vi "Get Timing.vi"(8 "error in (no error)":errorcluster, 11 "RP I-V Driver in":refnum<class "RP I-V Driver.lvclass">) -> (0 "error out":errorcluster, 1 "Decimation":i32=1, 2 "Rate":dbl=125000000.0 format="%#_6pHz", 3 "RP I-V Driver out":refnum<class "RP I-V Driver.lvclass">)   [LabVIEW 2024, in "RP I-V Driver.lvclass"]
uses:
  RP I-V Driver.lvclass
  D:/GitHub/NHMFL_Core/Libraries/Red Pitaya/Red Pitaya Digitizer/Red Pitaya Digitizer.lvclass
  Red Pitaya Digitizer/Red Pitaya Digitizer.lvclass/Red Pitaya Digitizer.ctl
  Red Pitaya Digitizer/Read Logic tag.vi
  Red Pitaya Digitizer/Red Pitaya Digitizer.lvclass
  RP I-V Driver.lvclass/RP I-V Driver.ctl
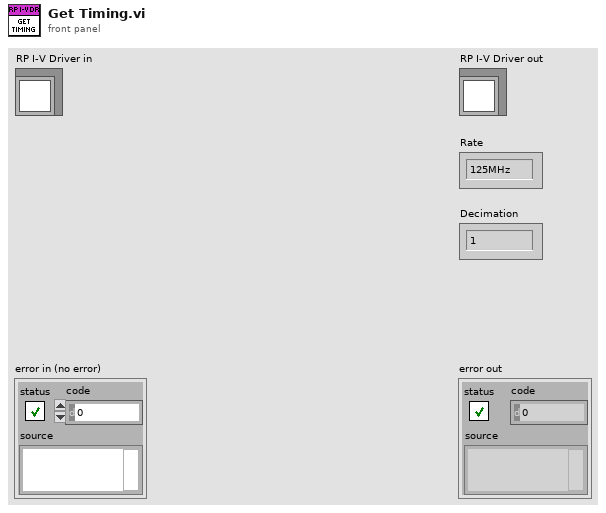
[diagram p1: front panel]
types:
  T1 = typedef "RP I-V Configuration.ctl" = cluster{"I-V parameters":T2, "Ranges":dbl[], "Post-trigger delay":dbl, "Post-trigger duration":dbl, "Output delay":dbl}
  T2 = typedef "I-V parameters.ctl" = cluster{"Start magnitude":dbl, "Magnitude increment":dbl, "End magnitude":dbl, "Ramp length":i32, "Top  length":i32, "Threshold ":dbl, "Processing delay":u16, "Output gain ":dbl, "Interpolation":i32, "Stop after":u16, "Detector window":i32}
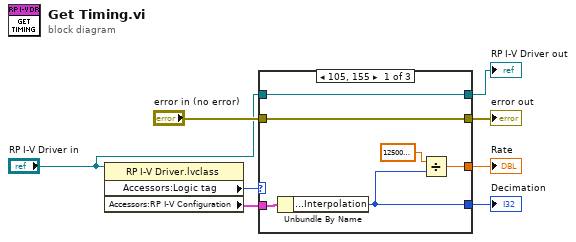
[diagram p0: block diagram]
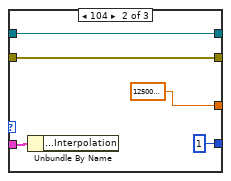
[diagram p2: hidden frame]
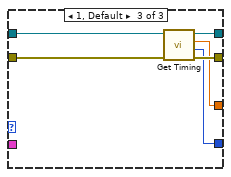
[diagram p3: hidden frame]
diagram:
  n1 = property class="RP I-V Driver.lvclass"(reference="RP I-V Driver in") -> ("Accessors:Logic tag"=w2:u16, "Accessors:RP I-V Configuration"=w1:T1)  [unwired: 1 in, 2 out]
  n2 = case shown="105, 155" w2 {
    tunnel: [w10 w18 w25] -> w8
    tunnel: [w11 1 ("Decimation") w24] -> w7
    tunnel: [w12 125000000.0 ("y") w23] -> w6
    tunnel: [w9 w17 w22] -> w5
    tunnel: "error in (no error)" -> [w10 w18 w21]
    tunnel: "RP I-V Driver in" -> [w9 w17 w20]
    tunnel: w1 -> [w14 w19 _]
    frame 105, 155 {
      n3 = Unbundle By Name(w14) -> ("I-V parameters.Interpolation"=w11:i32)
      n4 = Divide(x=125000000.0 ("y"), y=w11) -> (x/y=w12:dbl)
    }
    frame 104 {
      n5 = Unbundle By Name(w19) -> ()  [unwired: 1 out]
    }
    frame 1, Default {
      n6 = call-parent "Get Timing.vi"("error in (no error)"=w21, "Red Pitaya Digitizer in"=w20) -> ("error out"=w25:errorcluster, "Decimation"=w24:i32, "Rate"=w23:dbl, "Red Pitaya Digitizer out"=w22:refnum<class "RP I-V Driver.lvclass">)  [unwired: 6 in]
    }
  }
  "error out" <- w8
  "RP I-V Driver out" <- w5
  "Decimation" <- w7
  "Rate" <- w6
